vi "OC2 Read Response.vi"(4 "error in (no error)":errorcluster, 6 "Command":string, 7 "VISA resource name":refnum<visa-resource-name>) -> (0 "RX packet ok":bool, 1 "error out":errorcluster, 2 "output string":string, 3 "dup VISA resource name":refnum<visa-resource-name>)   [LabVIEW 2009]
doc: "TCM read response.vi\n\nLow Level VI that reads information from the TCM and performs checksum calculations\n\nCOPYRIGHT ELECTRON DYNAMICS LTD"
uses:
  <vilib>/Utility/error.llb/DialogType.ctl
panel:
  out "No of Bytes":u32
  out "read buffer":string
  # "Low level comms response"
  # "V1.02"
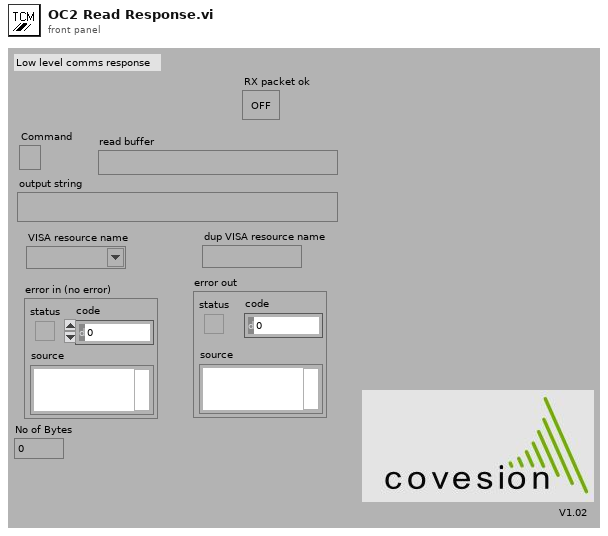
[diagram p1: front panel]
types:
  T1 = typedef "DialogType.ctl" = u16
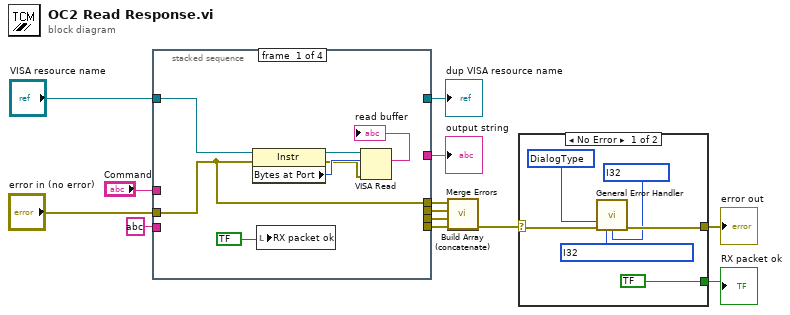
[diagram p0: block diagram]
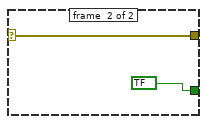
[diagram p2: hidden frame]
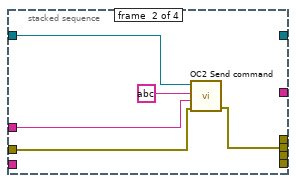
[diagram p3: hidden frame]
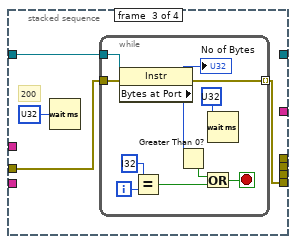
[diagram p4: hidden frame]
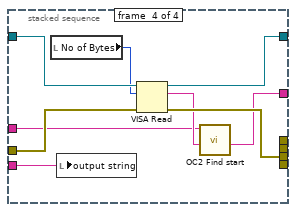
[diagram p5: hidden frame]
diagram:
  n1 = stacked-sequence {
    tunnel: [_ _ _ w43] -> w14
    tunnel: "VISA resource name" -> [w17 w24 w30 w46]
    tunnel: "error in (no error)" -> [w16 w23 w29 w45]
    tunnel: [_ _ _ w49] -> w9
    tunnel: [_ w25 _ _] -> w10
    tunnel: [_ _ _ w48] -> w12
    tunnel: [w16 _ _ _] -> w11
    tunnel: string ? ("output string") -> [_ _ _ w47]
    tunnel: [_ _ w28 _] -> w6
    tunnel: "Command" -> [_ w22 _ w41]
    frame #0 {
      n2 = property class="Instr"(reference=w17, error in=w16) -> (reference out=w20:refnum<visa-resource-name>, error out=w15:errorcluster, "Bytes at Port"=w19:u32)
      n3 = local write "RX packet ok"(bool ? ("Checksum ok")) -> ()
      n4 = VISA Read(VISA resource name=w20, byte count=w19, error in (no error)=w15) -> (read buffer=→"read buffer":string)  [unwired: 3 out]
    }
    frame #1 {
      n5 = call "OC2 Send command.vi"("VISA resource name"=w24, "Command data"=string ?, "Command"=w22, "error in (no error)"=w23) -> ("error out"=w25:errorcluster)  [unwired: 1 in, 1 out]
    }
    frame #2 {
      # "200"
      n6 = Wait (ms)(milliseconds to wait=u32 ?) -> ()  [unwired: 1 out]
      n7 = while {
        tunnel: w30 -> [w40]
        tunnel: w29 -> [w39]
        tunnel: [w38] -> w28 mode=indexing
        i -> [w36]
        stop <- w33 stop-if-true
        n8 = property class="Instr"(reference=w40, error in=w39) -> (error out=w38:errorcluster, "Bytes at Port"=w31:u32)  [unwired: 1 out]
        "No of Bytes" <- w31
        n9 = Equal?(x=i32 ?, y=w36) -> (x = y?=w35:bool)
        n10 = Greater Than 0?(x=w31) -> (x > 0?=w32:bool)
        n11 = Or(x=w32, y=w35) -> (x .or. y?=w33:bool)
        n12 = Wait (ms)(milliseconds to wait=u32 ?) -> ()  [unwired: 1 out]
      }
    }
    frame #3 {
      n13 = local read "No of Bytes"() -> (w44:u32)
      n14 = local write "output string"(w47) -> ()
      n15 = VISA Read(VISA resource name=w46, byte count=w44, error in (no error)=w45) -> (VISA resource name out=w48:refnum<visa-resource-name>, read buffer=w42:string, error out=w49:errorcluster)  [unwired: 1 out]
      n16 = call "OC2 Find start.vi"("input string"=w42, "Command"=w41) -> ("substring"=w43:string)  [unwired: 9 in]
    }
  }
  "output string" <- w14
  "dup VISA resource name" <- w12
  n17 = Build Array (concatenate)(w11, w10, w9, w6) -> (w1:errorcluster[])
  n18 = call <vilib>:"Merge Errors.vi"("error array in"=w1) -> ("error out"=w3:errorcluster)  [unwired: 6 in]
  n19 = case shown="No Error" w3 {
    selector: w3 -> [w54 w56]
    tunnel: [bool ? bool ?] -> w8
    tunnel: [w53 w56] -> w4
    frame #0 {
      w51 = T1 ? items=["no dialog", "OK message", "continue or stop message", "OK message + warnings", "continue/stop + warnings"] ("type of dialog (OK msg:1)")
      w52 = i32 ? items=["no exception", "cancel error on match", "set error on match"] ("[exception action] (none:0)")
      n20 = call <vilib>:"General Error Handler.vi"("type of dialog (OK msg:1)"=w51, "error in (no error)"=w54, "[exception action] (none:0)"=w52, "[exception code]"=i32 ? ("[error code] (0)")) -> ("error out"=w53:errorcluster)  [unwired: 7 in, 4 out]
    }
    frame #1 {
    }
  }
  "error out" <- w4
  "RX packet ok" <- w8
